vi "collatzSequence.vi"() -> ()   [LabVIEW 2024]
panel:
  out "grad-array":u64[](array[numeric])
  out "error out":errorcluster
  in  "error in (no error)":errorcluster
  in  "n":i32
  in  "g0":u64
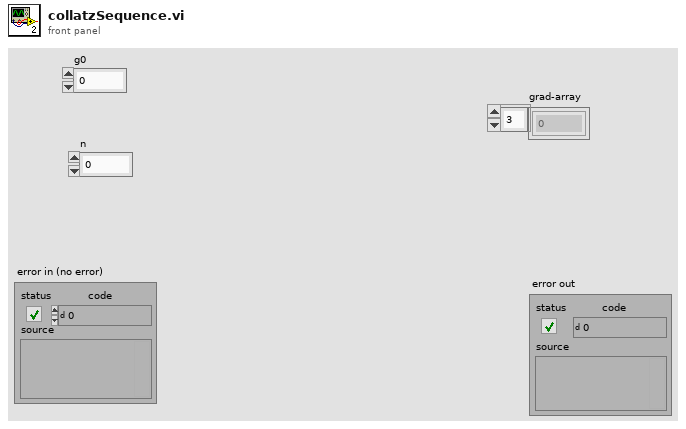
[diagram p1: front panel]
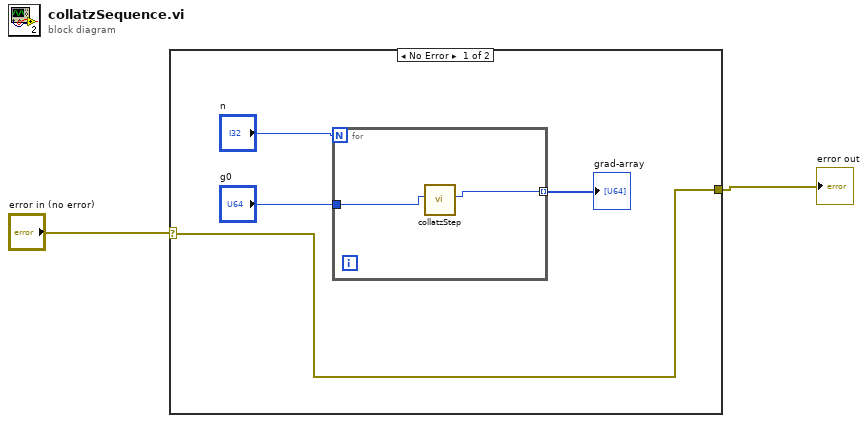
[diagram p0: block diagram]
diagram:
  n1 = case shown="No Error" "error in (no error)" {
    selector: "error in (no error)" -> [w3 w9]
    tunnel: [w3 w9] -> w1
    frame No Error {
      n2 = for {
        N: "n" -> [_]
        tunnel: "g0" -> [w8]
        tunnel: [w7] -> w4 mode=indexing
        n3 = call "collatzStep.vi"("gradn"=w8) -> ("gradnext"=w7:u64)  [unwired: 10 in]
      }
      "grad-array" <- w4
    }
    frame Error {
    }
  }
  "error out" <- w1
